vi "RemoveDuplicateTags.vi"(11 "Tags":string) -> (1 "Tag string":string, 3 "Tags out":string[](array[string]))   [LabVIEW 2022 SP3]
uses:
  <vilib>/Utility/error.llb/Trim Whitespace One-Sided.vi
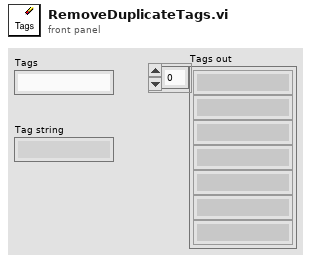
[diagram p1: front panel]
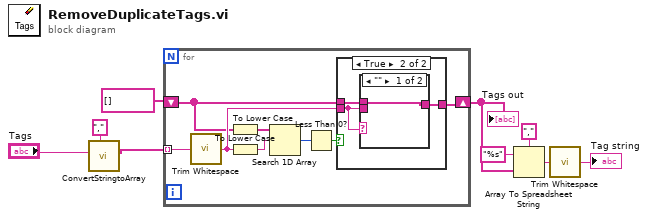
[diagram p0: block diagram]
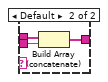
[diagram p3: hidden frame]
diagram:
  n1 = call "ConvertStringtoArray.vi"("delimiter (Tab)"=",", "Filter"="Tags") -> ("Array"=w3:string[])  [unwired: 9 in]
  n2 = for {
    tunnel: w3 -> [w14] mode=indexing
    shift-right: [w11] -> w7
    shift-left: string[] [] -> [w10]
    n3 = call <vilib>:"Trim Whitespace.vi"("string"=w14) -> ("trimmed string"=w12:string)  [unwired: 1 in]
    n4 = To Lower Case(string=w10) -> (all lower case string=w17:string[])
    n5 = To Lower Case(string=w12) -> (all lower case string=w16:string)
    n6 = Search 1D Array(1D array=w17, element=w16) -> (index of element=w15:i32)  [unwired: 1 in]
    n7 = Less Than 0?(x=w15) -> (x < 0?=w13:bool)
    n8 = case shown="True" w13 {
      tunnel: w10 -> [w18 w21]
      tunnel: w12 -> [_ w19]
      tunnel: [w18 w20] -> w11
      frame False {
      }
      frame True {
        n9 = case shown="\"\"" w19 {
          tunnel: w21 -> [w22 w25]
          tunnel: w19 -> [_ w24]
          tunnel: [w22 w23] -> w20
          frame "" {
          }
          frame Default {
            n10 = Build Array (concatenate)(w25, w24) -> (w23:string[])
          }
        }
      }
    }
  }
  "Tags out" <- w7
  n11 = Array To Spreadsheet String(delimiter (Tab)=",", array=w7, 3:"%s" ("format string")) -> (spreadsheet string=w2:string)
  n12 = call <vilib>:"Trim Whitespace.vi"("string"=w2) -> ("trimmed string"=→"Tag string":string)  [unwired: 1 in]
